vi "Global - Device Tree Items - NLHQ.vi"() -> ()   [LabVIEW 2015]
panel:
  out "device tree items":T1(array[cluster])=[{"Left Cell String"="NI cRIO (192.168.18.132)", "Child Text"=[], "Child Tag"="NI cRIO", "Item Indent"=0, "Child Only?"=FALSE, "Glyph Index"=1}, {"Left Cell String"="Mod1 (Slot1 NI 9239)", "Child Text"=[], "Child Tag"="Mod1", "Item Indent"=1, "Child Only?"=FALSE, "Glyph Index"=3}, {"Left Cell String"="NLHQ-X-02-A01", "Child Text"=[], "Child Tag"="NLHQ-X-02-A01", "Item Indent"=2, "Child Only?"=TRUE, "Glyph Index"=4}, {"Left Cell String"="NLHQ-X-04-A01", "Child Text"=[], "Child Tag"="NLHQ-X-04-A01", "Item Indent"=2, "Child Only?"=TRUE, "Glyph Index"=4}, {"Left Cell String"="NLHQ-X-04-A02", "Child Text"=[], "Child Tag"="NLHQ-X-04-A02", "Item Indent"=2, "Child Only?"=TRUE, "Glyph Index"=4}, {"Left Cell String"="NLHQ-X-06-A01", "Child Text"=[], "Child Tag"="NLHQ-X-06-A01", "Item Indent"=2, "Child Only?"=TRUE, "Glyph Index"=4}, {"Left Cell String"="Mod2 (Slot2 NI 9219)", "Child Text"=[], "Child Tag"="Mod2", "Item Indent"=1, "Child Only?"=FALSE, "Glyph Index"=3}, {"Left Cell String"="NLHQ-X-02-S01", "Child Text"=[], "Child Tag"="NLHQ-X-02-S01", "Item Indent"=2, "Child Only?"=TRUE, "Glyph Index"=4}, {"Left Cell String"="NLHQ-X-02-S02", "Child Text"=[], "Child Tag"="NLHQ-X-02-S02", "Item Indent"=2, "Child Only?"=TRUE, "Glyph Index"=4}, {"Left Cell String"="NLHQ-X-02-S03", "Child Text"=[], "Child Tag"="NLHQ-X-02-S03", "Item Indent"=2, "Child Only?"=TRUE, "Glyph Index"=4}, {"Left Cell String"="NLHQ-X-02-S04", "Child Text"=[], "Child Tag"="NLHQ-X-02-S04", "Item Indent"=2, "Child Only?"=TRUE, "Glyph Index"=4}, {"Left Cell String"="Mod3 (Slot3 NI 9219)", "Child Text"=[], "Child Tag"="Mod3", "Item Indent"=1, "Child Only?"=FALSE, "Glyph Index"=3}, {"Left Cell String"="NLHQ-X-03-S05", "Child Text"=[], "Child Tag"="NLHQ-X-03-S05", "Item Indent"=2, "Child Only?"=TRUE, "Glyph Index"=4}, {"Left Cell String"="NLHQ-X-03-S07", "Child Text"=[], "Child Tag"="NLHQ-X-03-S07", "Item Indent"=2, "Child Only?"=TRUE, "Glyph Index"=4}, {"Left Cell String"="NLHQ-X-03-S08", "Child Text"=[], "Child Tag"="NLHQ-X-03-S08", "Item Indent"=2, "Child Only?"=TRUE, "Glyph Index"=4}, {"Left Cell String"="NLHQ-X-03-S09", "Child Text"=[], "Child Tag"="NLHQ-X-03-S09", "Item Indent"=2, "Child Only?"=TRUE, "Glyph Index"=4}, {"Left Cell String"="Mod4 (Slot4 NI 9219)", "Child Text"=[], "Child Tag"="Mod4", "Item Indent"=1, "Child Only?"=FALSE, "Glyph Index"=3}, {"Left Cell String"="NLHQ-X-03-S04", "Child Text"=[], "Child Tag"="NLHQ-X-03-S04", "Item Indent"=2, "Child Only?"=TRUE, "Glyph Index"=4}, {"Left Cell String"="NLHQ-X-03-S06", "Child Text"=[], "Child Tag"="NLHQ-X-03-S06", "Item Indent"=2, "Child Only?"=TRUE, "Glyph Index"=4}, {"Left Cell String"="NLHQ-X-03-S10", "Child Text"=[], "Child Tag"="NLHQ-X-03-S10", "Item Indent"=2, "Child Only?"=TRUE, "Glyph Index"=4}, {"Left Cell String"="NLHQ-X-03-S11", "Child Text"=[], "Child Tag"="NLHQ-X-03-S11", "Item Indent"=2, "Child Only?"=TRUE, "Glyph Index"=4}, {"Left Cell String"="Mod5 (Slot5 NI 9219)", "Child Text"=[], "Child Tag"="Mod5", "Item Indent"=1, "Child Only?"=FALSE, "Glyph Index"=3}, {"Left Cell String"="NLHQ-X-05-S01", "Child Text"=[], "Child Tag"="NLHQ-X-05-S01", "Item Indent"=2, "Child Only?"=TRUE, "Glyph Index"=4}, {"Left Cell String"="NLHQ-X-05-S02", "Child Text"=[], "Child Tag"="NLHQ-X-05-S02", "Item Indent"=2, "Child Only?"=TRUE, "Glyph Index"=4}, {"Left Cell String"="NLHQ-X-05-S03", "Child Text"=[], "Child Tag"="NLHQ-X-05-S03", "Item Indent"=2, "Child Only?"=TRUE, "Glyph Index"=4}, {"Left Cell String"="NLHQ-X-05-S04", "Child Text"=[], "Child Tag"="NLHQ-X-05-S04", "Item Indent"=2, "Child Only?"=TRUE, "Glyph Index"=4}, {"Left Cell String"="Mod6 (Slot6 NI 9219)", "Child Text"=[], "Child Tag"="Mod6", "Item Indent"=1, "Child Only?"=FALSE, "Glyph Index"=3}, {"Left Cell String"="NLHQ-X-03-S01", "Child Text"=[], "Child Tag"="NLHQ-X-03-S01", "Item Indent"=2, "Child Only?"=TRUE, "Glyph Index"=4}, {"Left Cell String"="NLHQ-X-03-S02", "Child Text"=[], "Child Tag"="NLHQ-X-03-S02", "Item Indent"=2, "Child Only?"=TRUE, "Glyph Index"=4}, {"Left Cell String"="NLHQ-X-03-S03", "Child Text"=[], "Child Tag"="NLHQ-X-03-S03", "Item Indent"=2, "Child Only?"=TRUE, "Glyph Index"=4}, {"Left Cell String"="NLHQ-X-03-S12", "Child Text"=[], "Child Tag"="NLHQ-X-03-S12", "Item Indent"=2, "Child Only?"=TRUE, "Glyph Index"=4}, {"Left Cell String"="Mod7 (Slot7 NI 9219)", "Child Text"=[], "Child Tag"="Mod7", "Item Indent"=1, "Child Only?"=FALSE, "Glyph Index"=3}, {"Left Cell String"="NLHQ-X-03-S13", "Child Text"=[], "Child Tag"="NLHQ-X-03-S13", "Item Indent"=2, "Child Only?"=TRUE, "Glyph Index"=4}, {"Left Cell String"="NLHQ-X-06-S01", "Child Text"=[], "Child Tag"="NLHQ-X-06-S01", "Item Indent"=2, "Child Only?"=TRUE, "Glyph Index"=4}, {"Left Cell String"="NLHQ-X-06-S02", "Child Text"=[], "Child Tag"="NLHQ-X-06-S02", "Item Indent"=2, "Child Only?"=TRUE, "Glyph Index"=4}, {"Left Cell String"="NLHQ-X-06-S03", "Child Text"=[], "Child Tag"="NLHQ-X-06-S03", "Item Indent"=2, "Child Only?"=TRUE, "Glyph Index"=4}, {"Left Cell String"="Mod8 (RS485 ICPCON 7005)", "Child Text"=[], "Child Tag"="Mod8", "Item Indent"=1, "Child Only?"=FALSE, "Glyph Index"=3}, {"Left Cell String"="NLHQ-X-03-T01", "Child Text"=[], "Child Tag"="NLHQ-X-03-T01", "Item Indent"=2, "Child Only?"=TRUE, "Glyph Index"=4}, {"Left Cell String"="NLHQ-X-03-T02", "Child Text"=[], "Child Tag"="NLHQ-X-03-T02", "Item Indent"=2, "Child Only?"=TRUE, "Glyph Index"=4}, {"Left Cell String"="NLHQ-X-03-T03", "Child Text"=[], "Child Tag"="NLHQ-X-03-T03", "Item Indent"=2, "Child Only?"=TRUE, "Glyph Index"=4}, {"Left Cell String"="NLHQ-X-03-T04", "Child Text"=[], "Child Tag"="NLHQ-X-03-T04", "Item Indent"=2, "Child Only?"=TRUE, "Glyph Index"=4}, {"Left Cell String"="NLHQ-X-03-T05", "Child Text"=[], "Child Tag"="NLHQ-X-03-T05", "Item Indent"=2, "Child Only?"=TRUE, "Glyph Index"=4}, {"Left Cell String"="NLHQ-X-03-T06", "Child Text"=[], "Child Tag"="NLHQ-X-03-T06", "Item Indent"=2, "Child Only?"=TRUE, "Glyph Index"=4}, {"Left Cell String"="NLHQ-X-03-T07", "Child Text"=[], "Child Tag"="NLHQ-X-03-T07", "Item Indent"=2, "Child Only?"=TRUE, "Glyph Index"=4}, {"Left Cell String"="NLHQ-X-03-T08", "Child Text"=[], "Child Tag"="NLHQ-X-03-T08", "Item Indent"=2, "Child Only?"=TRUE, "Glyph Index"=4}] caption="设备树项目"
  # "在Utility - Edit Device Tree Items.vi 中编辑树形控件并执行可改变本全局变量，更改全局变量后需将新数据设置为默认。"
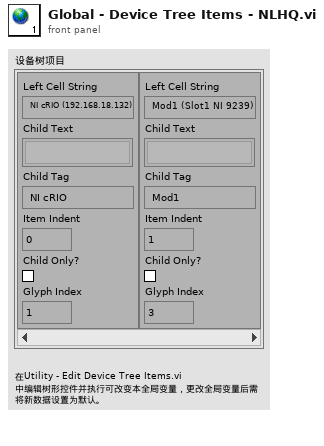
[diagram p1: front panel]
types:
  T1 = cluster{"Left Cell String":string, "Child Text":string[], "Child Tag":string, "Item Indent":i32, "Child Only?":bool, "Glyph Index":i32}[]
diagram:
